vi "K-ratio calc.vi"(0 "Desired Stripped mass":dbl, 1 "Current Molecular Mass":dbl, 2 "Desired Molecular Mass":dbl, 5 "Current Stripped Mass":dbl, 7 "Charge State":u8, 9 "Terminal Voltage":dbl, 11 "error in":errorcluster, 12 "PreAcc Voltage":dbl, 13 "Extractor Voltage":dbl) -> (4 "Kinetic energy ratio":dbl, 15 "error out":errorcluster)   [LabVIEW 2016, in "scale sub-VIs.lvlib"]
uses:
  sub-VIs/scale sub-VIs.lvlib
  <vilib>/imath/engines/lvmath2/RunTimeEngine/Managers/WorkSpace/UID Generator.vi
  <vilib>/imath/engines/lvmath2/RunTimeEngine/RunTimeType/NIMS_RunTimeType_From StrictType (excl LVString).vi
  <instcachedir>/0/NIMS_RunTimeType_From StrictType (excl LVString)_BBF44FB49F834B71AF7A14CCEDF8BECD.lvgen/NIMS_RunTimeType_From StrictType (excl LVString)_BBF44FB49F834B71AF7A14CCEDF8BECD_000.vi
  <vilib>/imath/engines/lvmath2/RunTimeEngine/LocalVariableDefStatement/MC_LocalVariableDefStatement_Display.vi
  <vilib>/imath/engines/lvmath2/RunTimeEngine/Managers/SymbolTable/Clear UID.vi
  <vilib>/imath/engines/lvmath2/RunTimeEngine/NodeEndStatement/NIMS_NodeEndStatement_Output.vi
  <instcachedir>/0/NIMS_NodeEndStatement_Output_53EC0D466D134D7ABD903AC30B43404B.lvgen/NIMS_NodeEndStatement_Output_53EC0D466D134D7ABD903AC30B43404B_001.vi
  <vilib>/imath/engines/lvmath2/RunTimeEngine/ErrorHandling/NIMS_Finalize Error.vi
  <vilib>/imath/engines/lvmath2/RunTimeEngine/Managers/SymbolTable/NIMS_WorkSpace.lvlib
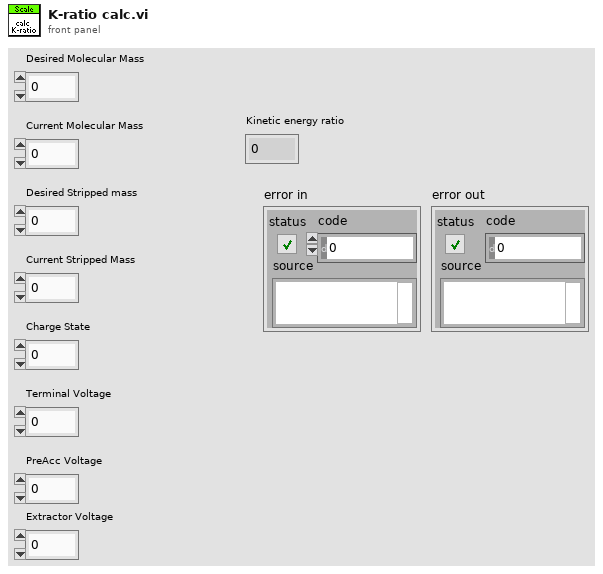
[diagram p1: front panel]
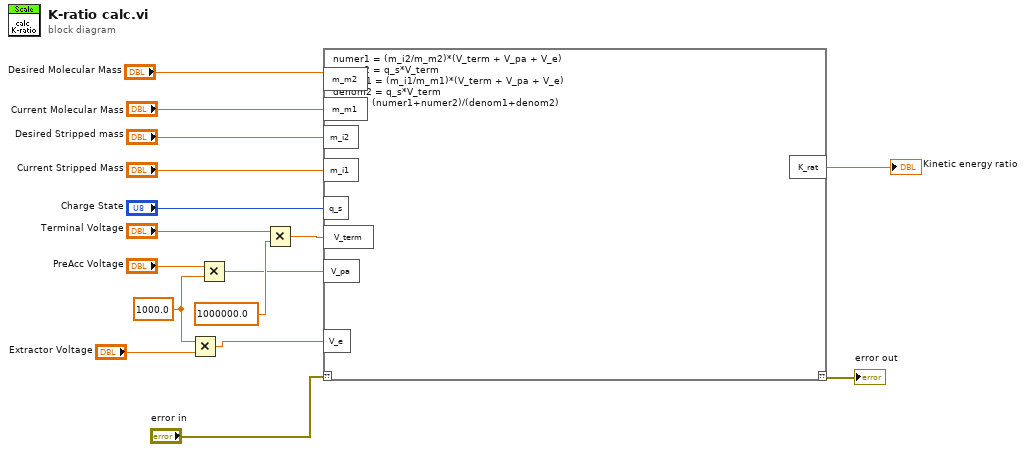
[diagram p0: block diagram]
diagram:
  w3 = 1000.0 ("y")
  n1 = Multiply(x=w3, y="Extractor Voltage") -> (x*y=w1:dbl)
  n2 = Multiply(x="PreAcc Voltage", y=w3) -> (x*y=w4:dbl)
  n3 = Multiply(x="Terminal Voltage", y=1000000.0) -> (x*y=w5:dbl)
  n4 = mathscript code="numer1 = (m_i2/m_m2)*(V_term + V_pa + V_e)\nnumer2 = q_s*V_term\ndenom1 = (m_i1/m_m1)*(V_term + V_pa + V_e)\ndenom2 = q_s*V_term\nK_rat = (numer1+numer2)/(denom1+denom2)"("??"="error in", "m_m2"="Desired Molecular Mass", "m_m1"="Current Molecular Mass", "m_i2"="Desired Stripped mass", "m_i1"="Current Stripped Mass", "q_s"="Charge State", "V_term"=w5, "V_pa"=w4, "V_e"=w1) -> ("??"=→"error out":errorcluster, "K_rat"=→"Kinetic energy ratio":dbl)
